vi "Advanced Cut - Build Snippet Path.vi"(8 "error in (no error)":errorcluster, 9 "Snippet Suffix":string, 10 "Original File Name":string, 11 "Destination Directory":path) -> (0 "error out":errorcluster, 3 "Snippet Path":path)   [LabVIEW 2016]
uses:
  <userlib>/_OpenG.lib/file/file.llb/Strip Path Extension - Path__ogtk.vi
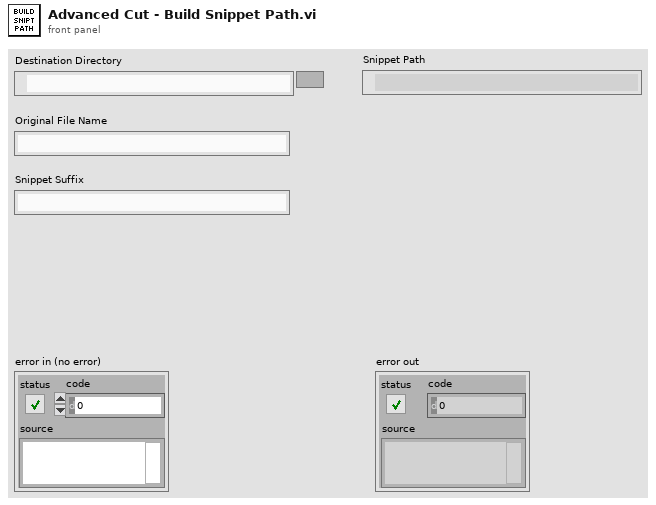
[diagram p1: front panel]
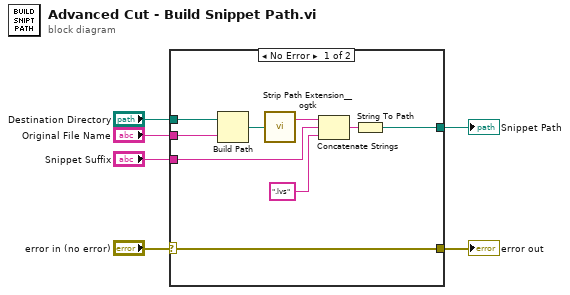
[diagram p0: block diagram]
diagram:
  n1 = case shown="No Error" "error in (no error)" {
    selector: "error in (no error)" -> [w7 w16]
    tunnel: "Destination Directory" -> [w11 _]
    tunnel: "Original File Name" -> [w10 _]
    tunnel: "Snippet Suffix" -> [w9 _]
    tunnel: [w8 _] -> w2
    tunnel: [w7 w16] -> w1
    frame No Error {
      n2 = Build Path(base path=w11, name or relative path=w10) -> (appended path=w12:path)
      n3 = call-poly <userlib>:"Strip Path Extension__ogtk.vi"("path"=w12) -> ("root"=w13:string)  [unwired: 1 out]
      n4 = Concatenate Strings(w13, w9, ".lvs") -> (w15:string)
      n5 = String To Path(string=w15) -> (path=w8:path)
    }
    frame Error {
    }
  }
  "error out" <- w1
  "Snippet Path" <- w2
